vi "Robot Global Data.vi"() -> ()   [LabVIEW 2013]
doc: "This global VI can contain as many global variables as you need. Place a control on the panel, give it a good name. To read or write to it from a VI, drag the icon to the diagram of that VI. You can also drag from the project. Click on the node to change which global you access. You shouldn't have multiple locations writing to a global or it will cause a race-condition."
uses:
  <vilib>/Rock Robotics/WPI/Camera/WPI_CameraImageSize.ctl
  <vilib>/Rock Robotics/WPI/DriverStation/WPI_DriverStationRobotMode2.ctl
  <vilib>/Rock Robotics/WPI/Joystick/WPI_JoystickButtonState.ctl
panel:
  in  "WinchButPressed":bool
  in  "WinchCase":dbl=1.5
  in  "Sorted Array":string[](array[string])
  in  "ManualControl":bool
  in  "CamFireReady":bool
  out "CamPower":dbl
  in  "CamOutGearPos":dbl=1.5
  in  "CamInGearPos":dbl=1.5
  in  "CamPos":dbl=1.5
  in  "CamFire":bool
  out "Harvester POT":dbl
  out "HarvRoller":dbl
  out "HarvPower":dbl
  in  "LimitSwitchIn":bool
  in  "LimitSwitchOut":bool
  in  "InButton":bool
  in  "OutButton":bool
  in  "HarvInPos":dbl=1.5
  in  "HarvOutPos":dbl=3.0
  in  "HarvPot":dbl
  in  "WinchPower":dbl=0.75
  in  "Buttons":T1
  in  "SetPointArray":dbl[](array[numeric])=[1.0, 2.0, 3.0]
  in  "Winch Pot Location":dbl
  out "Winch Motor Power Out":dbl
  out "Encoder":dbl
  out "Auton Array":dbl[][](array[numeric]) format="%0.3f"
  out "Current File":dbl
  out "Auton Files":string[](array[string])
  out "Number of Auton Files":dbl
  in  "Robot Mode":T2
  in  "LED toggle rate (ms)":u32=20
  in  "image size":T3=enum."320x240"
  in  "Enable Vision":bool
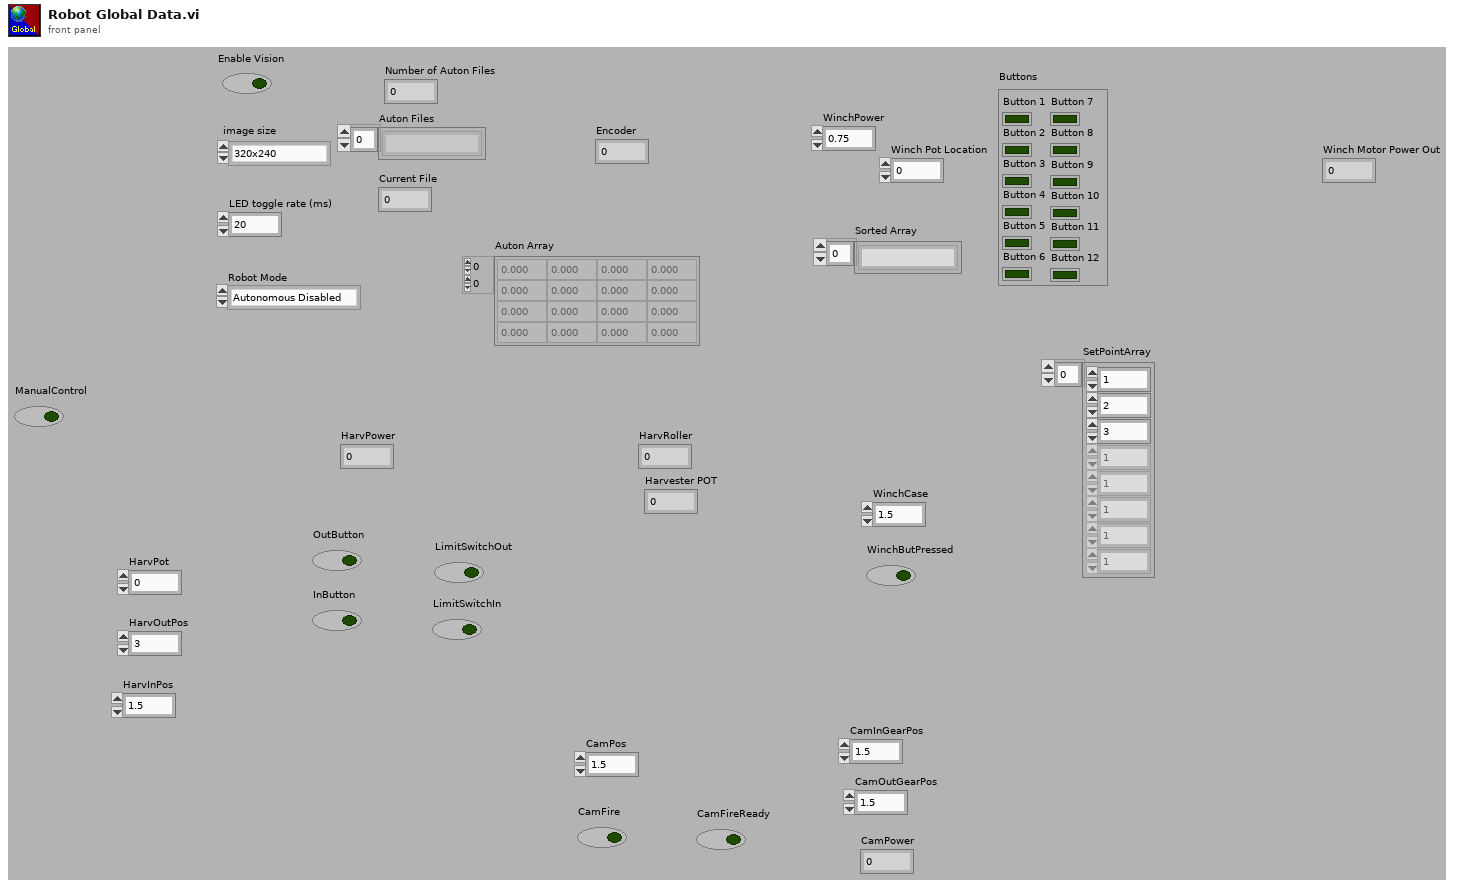
[diagram p1: front panel]
types:
  T1 = typedef "WPI_JoystickButtonState.ctl" = cluster{"Button 1":bool, "Button 2":bool, "Button 3":bool, "Button 4":bool, "Button 5":bool, "Button 6":bool, "Button 7":bool, "Button 8":bool, "Button 9":bool, "Button 10":bool, "Button 11":bool, "Button 12":bool}
  T2 = typedef "WPI_DriverStationRobotMode2.ctl" = enum16{"Autonomous Disabled", "Autonomous Enabled", "Teleop Disabled", "Teleop Enabled", "Timeout", "Finish", "Test Disabled", "Test Enabled"}
  T3 = typedef "WPI_CameraImageSize.ctl" = enum16{"640x480", "320x240", "160x120"}
diagram:
